vi "ex_subFileWrite.vi"(0 "Signals":dynamicdata(waveform), 1 "error in (no error)":errorcluster, 3 "Comment":string, 4 "Enable":bool=TRUE, 6 "new_file":bool, 7 "File Path in":path=path "c:/testdata.txt", 8 "File Dialog":bool, 9 "column headings":enum32{"one per segment", "once", "none"}(radio), 10 "Description":string, 11 "x_columns":enum32{"none", "one", "multiple"}(radio)=enum."multiple", 12 "multi_file":bool, 13 "fixed_width":bool=TRUE, 14 "serno_digits":i32=3, 15 "time_format_string":string="%Y-%m-%d_%H%M%S", 16 "overwrite_mode_multi":T6(ring)=enum."overwrite & backup", 17 "new_file_mode":u16(ring)=1 items=["Date & Time", "Serial No.", "Both"], 18 "overwrite_mode":T1(radio)=enum."overwrite & backup", 19 "new file options":T5, 20 "delimiter":string="\t", 22 "Reset":bool, 23 "Static File Path in":path=path "c:/testdata.txt", 24 "Lock file":bool, 25 "Simulate Non-First Call":bool, 26 "storage_format":T2, 27 "Ask each iteration":bool) -> (2 "error out":errorcluster, 5 "File Path out":path, 21 "Saving Data":bool)   [LabVIEW 2020]
uses:
  ex_NewFileOptions.ctl
  ex_WriteFileParams.ctl
  express input/ExFileReadBlock.llb/ex_ReadFileParams.ctl
  express shared/ExFile.llb/ex_FileFormats.ctl
panel:
  out "previous path":path
  in  "file params":T3={"delimiter"="\t", "origin time"=timestamp(0 s since 1904-01-01), "Flags"={"include col headings?"=TRUE, "x_columns"=0, "col headings always?"=TRUE, "time preference"=0, "hide col headings"=FALSE}, "Decimal Separator"=""} {"Flags"."time preference" items=["Absolute", "Relative"]; "Flags"."x_columns" items=["None", "One", "Multiple"]; "origin time" format="%<%X\n%x>T"}
  in  "1st":bool
  in  "File refnum":refnum<file>
  in  "origin time":timestamp format="%<%I:%M:%S %p\n%m/%d/%Y>T"
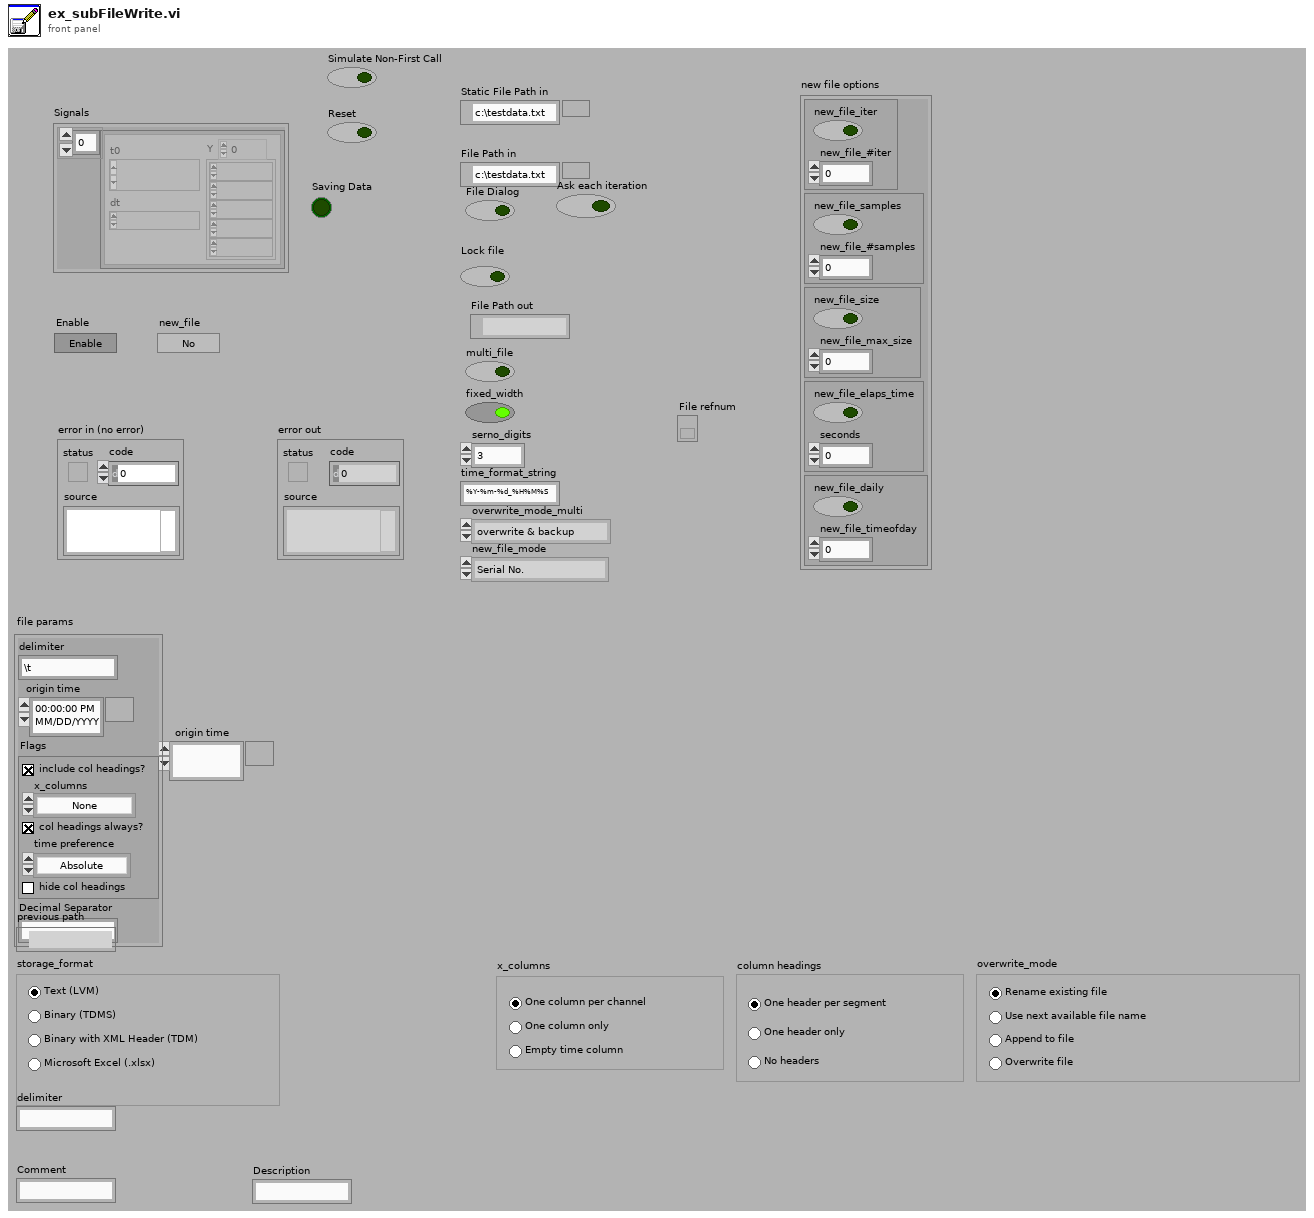
[diagram p1: front panel]
types:
  T1 = enum32{"overwrite", "overwrite & backup", "append", "next avail"}
  T2 = typedef "ex_FileFormats.ctl" = enum32{"lvm", "tdm", "tdms", "xlsx"}
  T3 = typedef "ex_WriteFileParams.ctl" = cluster{"delimiter":string, "origin time":timestamp, "Flags":T4, "Decimal Separator":string}
  T4 = typedef "ex_ReadFileParams.ctl" = cluster{"include col headings?":bool, "x_columns":u16, "col headings always?":bool, "time preference":u16, "hide col headings":bool}
  T5 = typedef "ex_NewFileOptions.ctl" = cluster{cluster{"new_file_iter":bool, "new_file_#iter":i32}, cluster{"new_file_samples":bool, "new_file_#samples":i32}, cluster{"new_file_size":bool, "new_file_max_size":i32}, cluster{"new_file_elaps_time":bool, "seconds":i32}, cluster{"new_file_daily":bool, "new_file_timeofday":i32}}
  T6 = enum16{"overwrite", "overwrite & backup", "next avail"}
  T7 = typedef "ex_userdefproperties.ctl" = cluster{"DAQmx Task":refnum<k21>, "User-defined properties":T8[], "Live values":variant[]}
  T8 = typedef "ex_userDefProperty.ctl" = cluster{"Name":string, "Object type":string, "usiDataType":T9, "propertySourceType":T10, "propertySource":string, "Value":variant, "ID":i32, "use def name":bool, "Source":string, "Built-in Prop":bool, "Attribute Type Enum":string[]}
  T9 = typedef "usiDataType.ctl" = enum16{"eNoTypeUsi", "eInt8Usi", "eInt16Usi", "eInt32Usi", "eInt64Usi", "eUInt8Usi", "eUInt16Usi", "eUInt32Usi", "eUInt64Usi", "eFloat32Usi", "eFloat64Usi", "- 0", "- 1", "- 2", "- 3", "- 4", "- 5", "- 6", "- 7", "- 8", "- 9", "eString8Usi", "eString16Usi", "eStringUsi", "eEnumUsi", "- 10", "- 11", "- 12", "- 13", "- 14", "eTimeUsi", "- 15", "- 16", "- 17", "- 18", "- 19", "- 20", "- 21", "- 22", "- 23", "eInstanceUsi", "eStoreUsi"}
  T10 = typedef "ex_propertySource.ctl" = enum16{"Manual", "System", "DAQmx Channel", "Terminal", "Ignore"}
  T11 = cluster{"file params":T3, "column headings":enum32{"one per segment", "once", "none"}, "origin time":timestamp, "File refnum":refnum<file>, "overwrite_mode_multi":enum16{"overwrite", "overwrite & backup", "next avail"}, "overwrite_mode":enum32{"overwrite", "overwrite & backup", "append", "next avail"}, "File Dialog":bool, "Description Out":string, "Comment Out":string, "serno_digits":i32, "fixed_width":bool, "new_file_mode":u16, "time_format_string":string, "multi_file":bool, "new file options":T5, "new_file":bool, "Simulate Non-First Call":bool}
  T12 = cluster{"channel\nrefnums":refnum<k20>[], "channel names":string[], "channel types":string[], "file refnum":refnum<k20>, "group refnum":refnum<k20>, "group name":string, "group type":string, "next T0":timestamp[], "dT":dbl[], "Start Time Stamp":timestamp, "channel length":u32[], "group index":u32, "group refnums":refnum<k20>[], "file name":string, "segment index":u32}
  T13 = typedef "ex_appendInfoTDM.ctl" = cluster{"channel\nrefnums":refnum<k20>[], "channel names":string[], "channel types":string[], "file refnum":refnum<k20>, "group refnum":refnum<k20>, "group name":string, "group type":string, "next T0":timestamp[], "dT":dbl[], "Start Time Stamp":timestamp, "channel length":u32[], "group index":u32, "group refnums":refnum<k20>[], "file name":string, "segment index":u32}
  T14 = cluster{"Start Timestamp":timestamp, "Timestamp":timestamp, "Relative Time?":bool, "X Dimension":string, "Signal Name":string, "Y Units":string, "X0":timestamp, "dX":dbl, "nPoints":i32}[]
  T15 = typedef "ex_WaveformAttribsPlus.ctl" = cluster{"Start Timestamp":timestamp, "Timestamp":timestamp, "Relative Time?":bool, "X Dimension":string, "Signal Name":string, "Y Units":string, "X0":timestamp, "dX":dbl, "nPoints":i32}
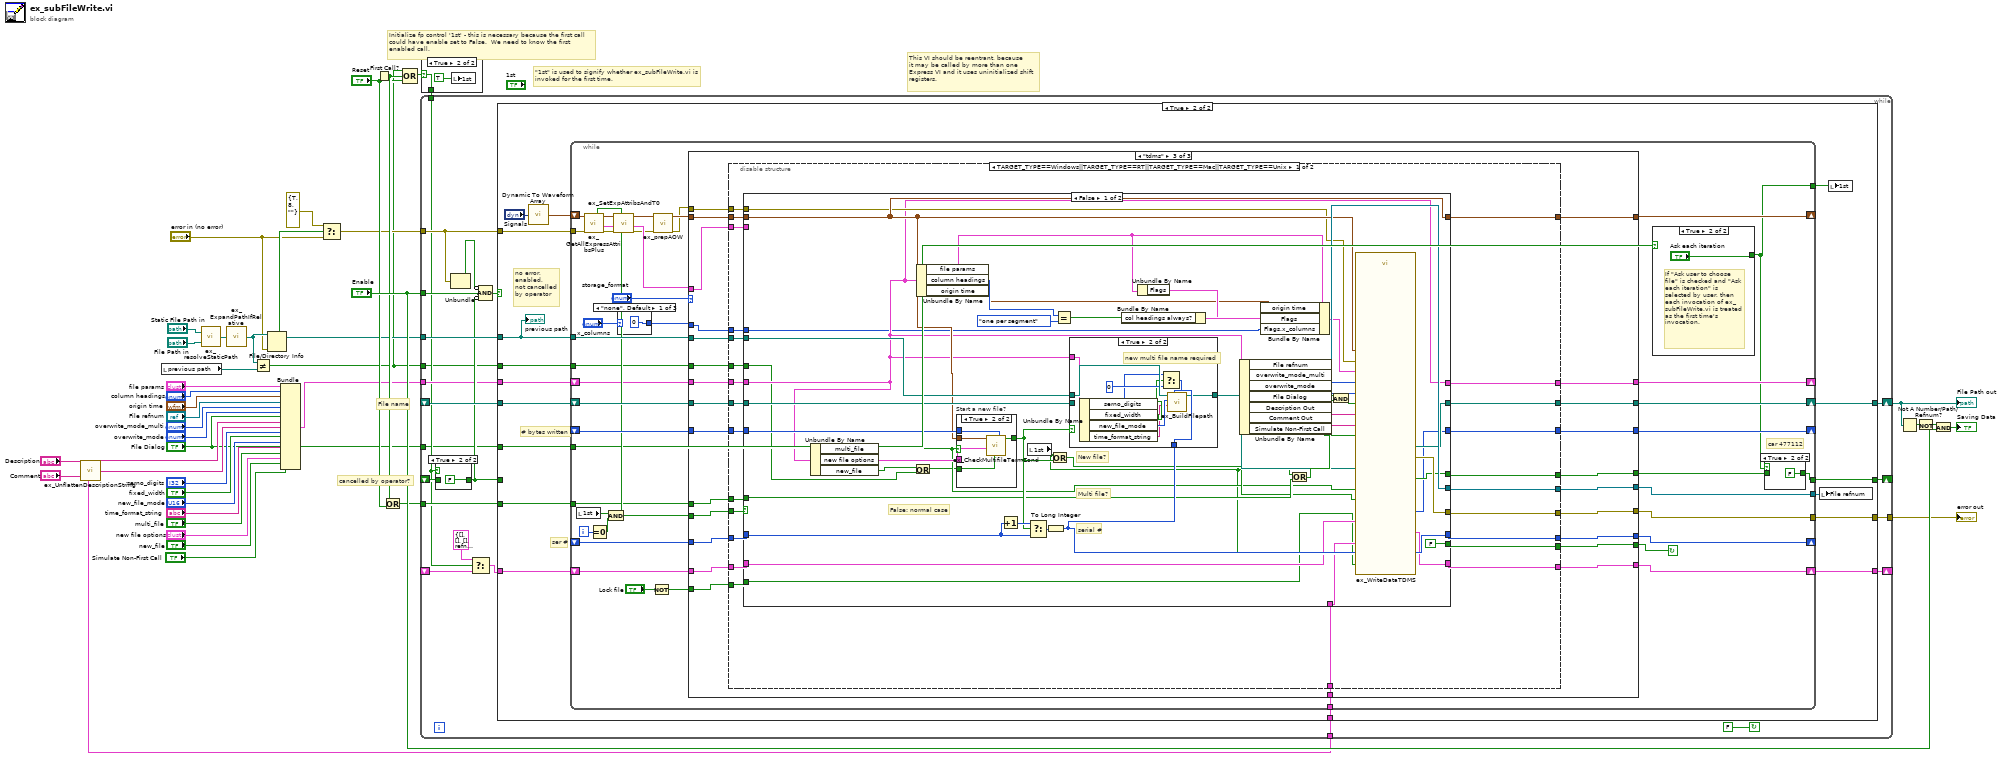
[diagram p0: block diagram]
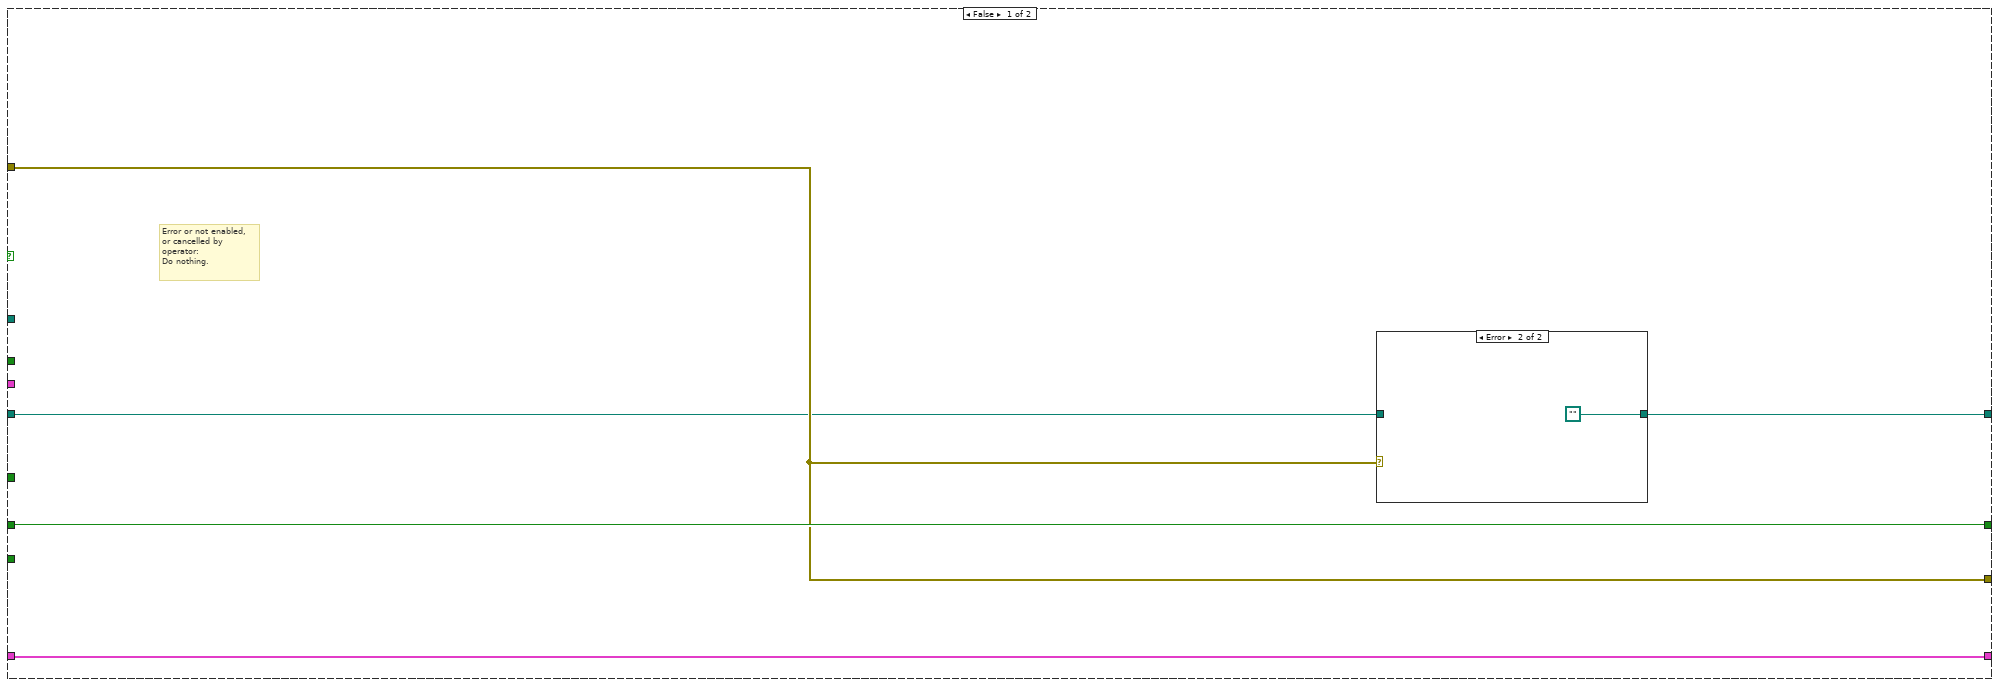
[diagram p3: hidden frame]
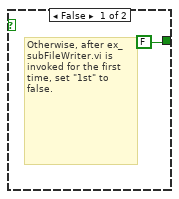
[diagram p6: hidden frame]
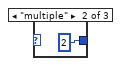
[diagram p7: hidden frame]
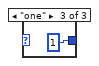
[diagram p8: hidden frame]
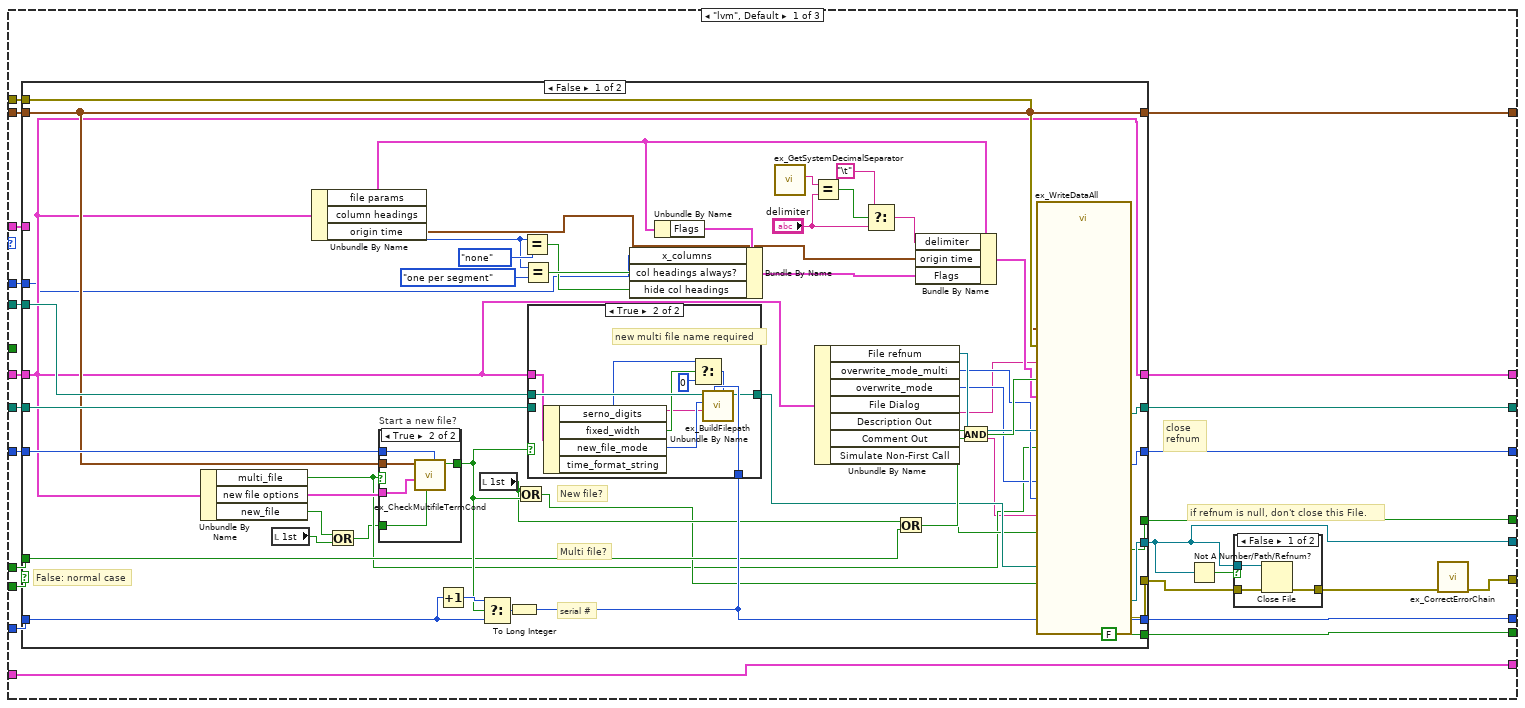
[diagram p9: hidden frame]
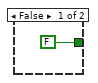
[diagram p12: hidden frame]
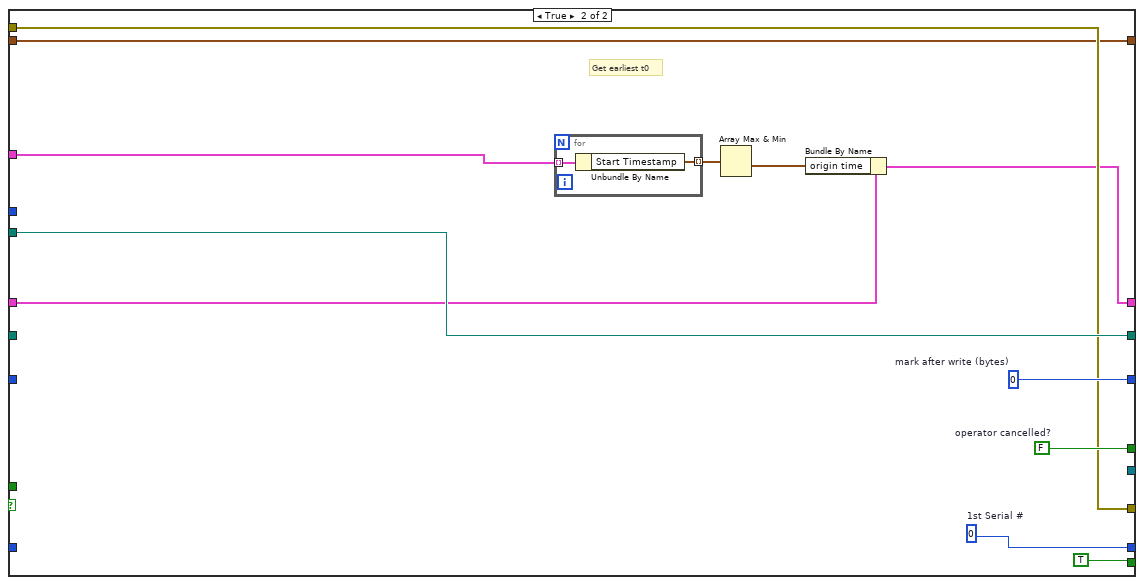
[diagram p13: hidden frame]
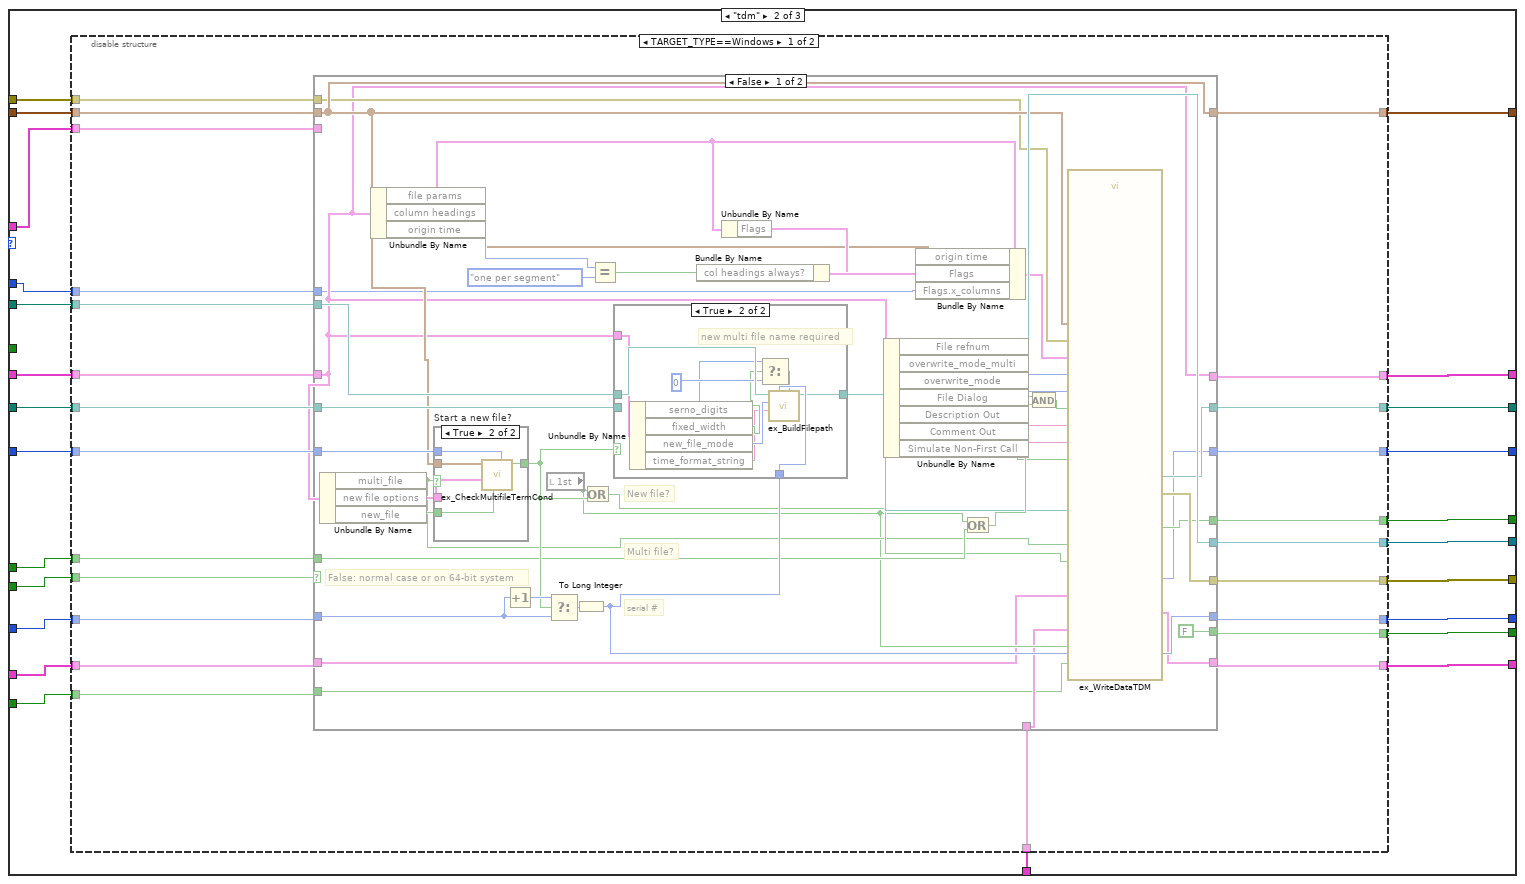
[diagram p14: hidden frame]
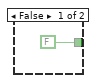
[diagram p16: hidden frame]
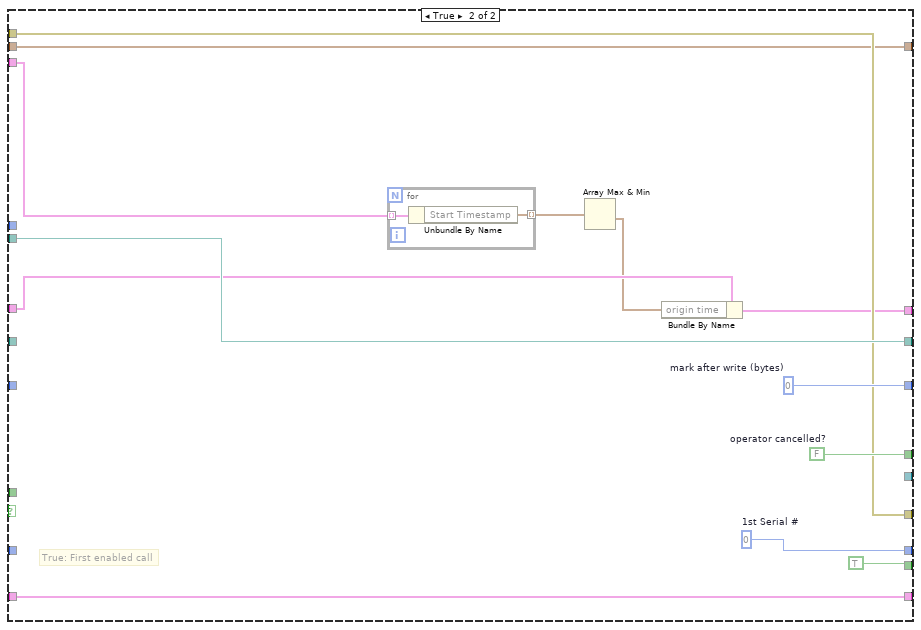
[diagram p17: hidden frame]
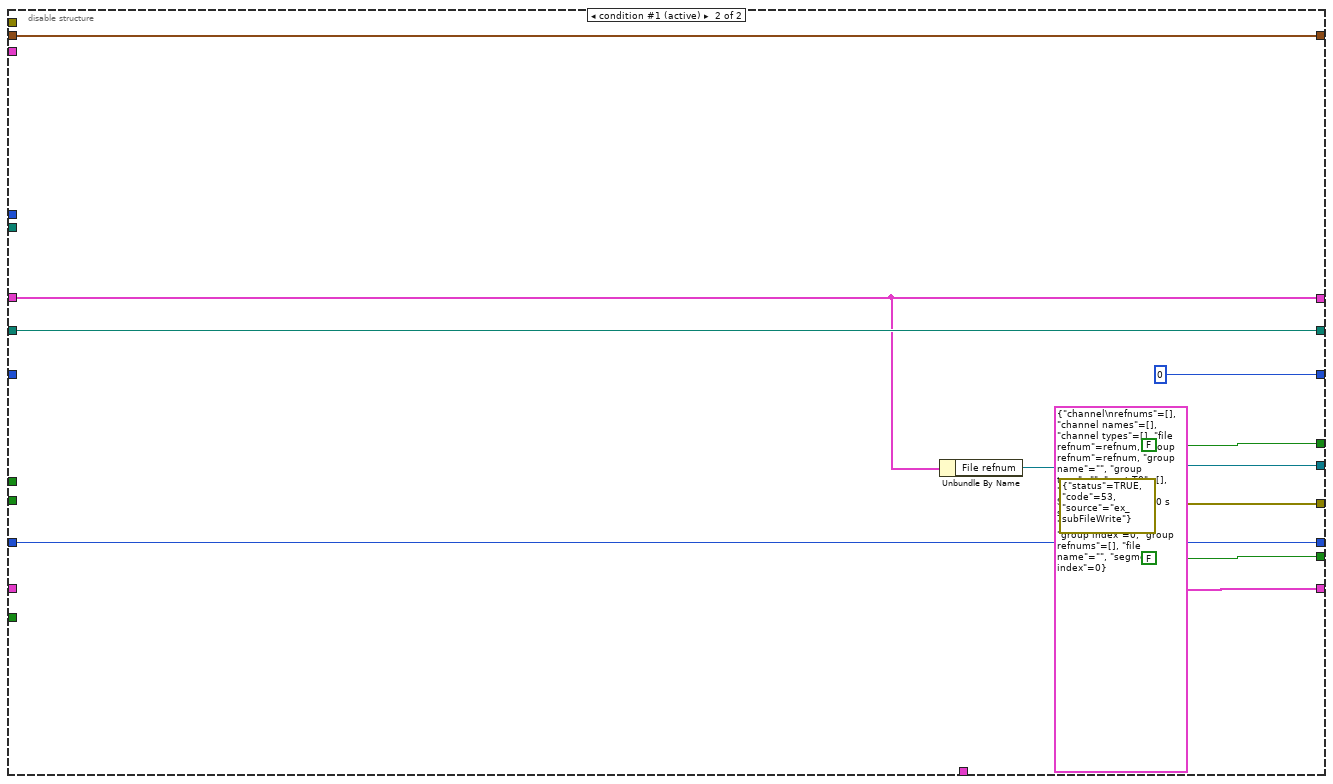
[diagram p18: hidden frame]
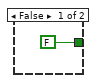
[diagram p20: hidden frame]
diagram:
  # "\"1st\" is used to signify whether ex_subFileWrite.vi is invoked for the first time."
  # "File name"
  # "This VI should be reentrant, because\nit may be called by more than one\nExpress VI and it uses uninitialized shift \nregisters."
  # "cancelled by operator?"
  # "Initialize fp control '1st' - this is necessary because the first call\ncould have enable set to False.  We need to know the first\nenabled call."
  n1 = call "ex_UnflattenDescriptionString.vi"("Description"="Description", "Comment"="Comment") -> ("Description Out"=w7:string, "Comment Out"=w6:string, "DAQmx Task"=w5:T7)
  n2 = local read "previous path"() -> (w36:path)
  n3 = call "ex_resolveStaticPath.vi"("file path in"="File Path in", "static path in"="Static File Path in") -> ("Path"=w14:path)
  n4 = call "ex_ExpandPathIfRelative.vi"("Path"=w14) -> ("Expanded path"=w13:path)  [unwired: 4 out]
  n5 = Not Equal?(x=w13, y=w36) -> (x != y?=w1:bool)
  n6 = File/Directory Info(path=w13, error in="error in (no error)") -> (path out=w12:path, directory=w10:bool)  [unwired: 5 out]
  n7 = Bundle("file params"="file params", "column headings"="column headings", "origin time"="origin time", "File refnum"="File refnum", "overwrite_mode_multi"="overwrite_mode_multi", "overwrite_mode"="overwrite_mode", "File Dialog"="File Dialog", "Description Out"=w7, "Comment Out"=w6, "serno_digits"="serno_digits", "fixed_width"="fixed_width", "new_file_mode"="new_file_mode", "time_format_string"="time_format_string", "multi_file"="multi_file", "new file options"="new file options", "new_file"="new_file", "Simulate Non-First Call"="Simulate Non-First Call") -> (w15:T11)  [unwired: 1 out]
  n8 = Select(t=errorcluster {"status"=TRUE, "code"=8, "source"=""}, s=w10, f="error in (no error)") -> (s? t:f=w11:errorcluster)
  n9 = First Call?() -> (First Call?: T/F=w34:bool)
  n10 = Or(x=w34, y="Reset") -> (x .or. y?=w32:bool)
  n11 = Compound Arithmetic op=OR(w1, w34, "Reset") -> (w35:bool)
  n12 = case shown="True" w35 {
    selector: w35 -> [w44 w45]
    tunnel: [w44 w45] -> w43
    frame False {
    }
    frame True {
      n13 = local write "1st"(TRUE ("1st")) -> ()
    }
  }
  n14 = while {
    tunnel: [w68] -> w31
    tunnel: w43 -> [w49]
    tunnel: w11 -> [w66]
    shift-right: [w64] -> _
    shift-left: _ -> [w63]
    shift-right: [w61] -> w30
    shift-left: _ -> [w62]
    tunnel: "Enable" -> [w60]
    tunnel: w12 -> [w59]
    tunnel: w32 -> [w56]
    tunnel: w15 -> [w55]
    shift-right: [w54] -> _
    shift-left: _ -> [w51]
    tunnel: w5 -> [w53]
    tunnel: "File Dialog" -> [w48]
    tunnel: w1 -> [w47]
    stop <- FALSE continue-if-true
    n15 = case shown="True" w49 {
      tunnel: w63 -> [w69 _]
      tunnel: [w69 FALSE ("operator cancelled?")] -> w57
      frame False {
      }
      frame True {
      }
    }
    n16 = Unbundle(w66) -> ("status"=w58:bool)  [unwired: 2 out]
    n17 = Select(t=T12 {"channel\nrefnums"=[], "channel names"=[], "channel types"=[], "file refnum"=refnum, "group refnum"=refnum, "group name"="", "group type"="", "next T0"=[], "dT"=[], "Start Time Stamp"=timestamp(0 s since 1904-01-01), "channel length"=[], "group index"=0, "group refnums"=[], "file name"="", "segment index"=0} ("append info out"), s=w49, f=w51) -> (s? t:f=w50:T13)
    n18 = Compound Arithmetic op=AND(invert w58, w60, invert w57) -> (w67:bool)
    n19 = case shown="True" w67 {
      tunnel: [w73 w85] -> w68
      tunnel: w66 -> [w73 w94]
      tunnel: [w75 w93] -> w64
      tunnel: w57 -> [w75 _]
      tunnel: [w72 w92] -> w61
      tunnel: w62 -> [w71 w91]
      tunnel: w59 -> [_ w82]
      tunnel: w56 -> [_ w89]
      tunnel: w55 -> [_ w87]
      tunnel: [w74 w84] -> w54
      tunnel: w50 -> [w74 w83]
      tunnel: w53 -> [_ w81]
      tunnel: w48 -> [_ w79]
      tunnel: w47 -> [_ w78]
      frame False {
        # "Error or not enabled,\nor cancelled by\noperator:\nDo nothing."
        n20 = case shown="Error" w73 {
          tunnel: [w76 path ""] -> w72
          tunnel: w71 -> [w76 _]
          frame No Error {
          }
          frame Error {
          }
        }
      }
      frame True {
        # "no error,\nenabled,\nnot cancelled\nby operator"
        # "# bytes written"
        # "ser #"
        n21 = call "Dynamic To Waveform Array.vi"("Input"="Signals") -> ("Output"=w86:waveform(dbl)[])  [unwired: 4 out]
        n22 = while {
          tunnel: w94 -> [w124]
          shift-right: [w133] -> _
          shift-left: _ -> [w132]
          tunnel: [w135] -> w85
          shift-right: [w125] -> w92
          shift-left: w91 -> [w131]
          shift-right: [w127] -> _
          shift-left: _ -> [w134]
          tunnel: [w130] -> w88
          tunnel: w82 -> [w126]
          tunnel: [w96] -> w93
          shift-right: [w123] -> _
          shift-left: w86 -> [w112]
          tunnel: w89 -> [w115]
          shift-right: [w111] -> _
          shift-left: w87 -> [w113]
          shift-right: [w110] -> w84
          shift-left: w83 -> [w109]
          tunnel: w81 -> [w102]
          tunnel: [w98] -> w80
          tunnel: w79 -> [w99]
          tunnel: w78 -> [w95]
          i -> [w129]
          stop <- w136 continue-if-true
          # "car 477112"
          n23 = local read "1st"() -> (w116:bool)
          n24 = call "ex_GetAllExpressAttribsPlus.vi"("error in"=w124, "Signals in"=w112) -> ("error out"=w118:errorcluster, "All Express Wave Attributes Plus"=w117:T14, "Signals out"=w121:waveform(dbl)[], "Time Attribs Not Found"=w119:bool[])  [unwired: 1 in, 5 out]
          n25 = Equal To 0?(x=w129) -> (x = 0?=w128:bool)
          n26 = And(x=w116, y=w128) -> (x .and. y?=w122:bool)
          n27 = call "ex_SetExpAttribsAndT0.vi"("Latch Origin TS? (T)"=w122, "Set? (T if empty)"=w119, "error in (no error)"=w118, "Express Attributes Plus in"=w117, "Signals"=w121) -> ("error out"=w104:errorcluster, "Express Wave Attributes Plus out"=w120:T15[], "Signals With Attributes"=w106:waveform(dbl)[])  [unwired: 1 in, 3 out]
          n28 = case shown="\"none\", Default" "x_columns" {
            tunnel: [u16 0 ("x_columns") u16 2 ("x_columns") u16 1 ("x_columns")] -> w107
            frame "none", Default {
            }
            frame "multiple" {
            }
            frame "one" {
            }
          }
          n29 = Not(x="Lock file") -> (.not. x?=w100:bool)
          n30 = call "ex_prepAOW.vi"("error in (no error)"=w104, "Dynamic Data"=w106) -> ("error out"=w103:errorcluster, 3:w105:waveform(dbl)[])  [unwired: 1 in, 3 out]
          n31 = case shown="\"tdms\"" "storage_format" {
            tunnel: [w167 w277 w413] -> w136
            tunnel: [w151 w276 w412] -> w135
            tunnel: w134 -> [w166 w275 w411]
            tunnel: [w165 w274 w410] -> w133
            tunnel: w132 -> [w164 w273 w409]
            tunnel: w131 -> [w163 w272 w408]
            tunnel: [w144 w261 w397] -> w130
            tunnel: [w162 w271 w407] -> w127
            tunnel: w126 -> [w161 w270 w406]
            tunnel: [w160 w269 w405] -> w97
            tunnel: [w159 w268 w404] -> w125
            tunnel: [w158 w267 w403] -> w123
            tunnel: w122 -> [w157 w266 w402]
            tunnel: w105 -> [w156 w260 w396]
            tunnel: w103 -> [w155 w265 w401]
            tunnel: w120 -> [w154 w264 w400]
            tunnel: w115 -> [w153 w263 w399]
            tunnel: w113 -> [w152 w262 w398]
            tunnel: [w150 w259 w395] -> w111
            tunnel: [w149 w258 w394] -> w110
            tunnel: w109 -> [w149 w257 w393]
            tunnel: w107 -> [w148 w256 w392]
            tunnel: w102 -> [_ w255 w391]
            tunnel: w100 -> [_ w254 w390]
            tunnel: w95 -> [_ _ w389]
            frame "lvm", Default {
              # "if refnum is null, don't close this File."
              # "close\nrefnum"
              n32 = case shown="False" w157 {
                tunnel: [FALSE TRUE] -> w167
                tunnel: [w195 _] -> w144
                tunnel: [w192 w244] -> w147
                tunnel: [w193 w251] -> w162
                tunnel: w166 -> [w215 _]
                tunnel: w155 -> [w211 w244]
                tunnel: [w220 w249] -> w165
                tunnel: [w194 w250] -> w159
                tunnel: w164 -> [w221 _]
                tunnel: w163 -> [w217 _]
                tunnel: w156 -> [w185 w243]
                tunnel: w161 -> [w214 w250]
                tunnel: [w186 w247] -> w160
                tunnel: w154 -> [_ w245]
                tunnel: [w185 w243] -> w158
                tunnel: w153 -> [w204 _]
                tunnel: w152 -> [w183 w242]
                tunnel: [w183 w240] -> w150
                tunnel: w148 -> [w182 _]
                frame False {
                  # "Multi file?"
                  # "New file?"
                  # "False: normal case"
                  # "serial #"
                  n33 = Unbundle By Name(w183) -> ("multi_file"=w187:bool, "new file options"=w196:T5, "new_file"=w174:bool)
                  n34 = local read "1st"() -> (w173:bool)
                  n35 = Unbundle By Name(w183) -> ("file params"=w202:T3, "column headings"=w201:enum32{"one per segment", "once", "none"}, "origin time"=w184:timestamp)
                  n36 = Or(x=w174, y=w173) -> (x .or. y?=w172:bool)
                  n37 = case "Start a new file?" shown="True" w187 {
                    tunnel: [FALSE ("start new file?") w239] -> w216
                    tunnel: w185 -> [_ w238]
                    tunnel: w215 -> [_ w237]
                    tunnel: w196 -> [_ w236]
                    tunnel: w172 -> [_ w235]
                    frame False {
                    }
                    frame True {
                      n38 = call "ex_CheckMultifileTermCond.vi"("file size (bytes)"=w237, "new_file_now"=w235, "termination conditions"=w236, "Signals"=w238) -> ("start new file?"=w239:bool)  [unwired: 7 out]
                    }
                  }
                  n39 = Increment(x=w221) -> (x+1=w222:i32)
                  n40 = local read "1st"() -> (w203:bool)
                  n41 = Select(t=w222, s=w216, f=w221) -> (s? t:f=w219:i32)
                  n42 = To Long Integer(number=w219) -> (32bit integer=w220:i32)
                  n43 = Or(x=w203, y=w216) -> (x .or. y?=w188:bool)
                  n44 = Equal?(x=w201, y=enum16{"one per segment", "once", "none"}."none") -> (x = y?=w207:bool)
                  n45 = Equal?(x=w201, y=enum16{"one per segment", "once", "none"}."one per segment") -> (x = y?=w208:bool)
                  n46 = case shown="True" w216 {
                    tunnel: w220 -> [_ w233]
                    tunnel: [w223 w232] -> w191
                    tunnel: w217 -> [w223 _]
                    tunnel: w214 -> [_ w231]
                    tunnel: w183 -> [_ w228]
                    frame False {
                      # "No new file - use old file name"
                    }
                    frame True {
                      # "new multi file name required"
                      n47 = Unbundle By Name(w228) -> ("serno_digits"=w227:i32, "fixed_width"=w226:bool, "new_file_mode"=w225:u16, "time_format_string"=w224:string)
                      n48 = Select(t=w227, s=w226, f=0) -> (s? t:f=w229:i32)
                      n49 = call "ex_BuildFilepath.vi"("serial digits"=w229, "serial num"=w233, "time format string"=w224, "naming mode"=w225, "name base"=w231) -> ("built name"=w232:path)  [unwired: 1 in, 5 out]
                    }
                  }
                  n50 = Unbundle By Name(w202) -> ("Flags"=w212:T4)
                  n51 = Bundle By Name(cluster=w212, "x_columns"=w182, "col headings always?"=w208, "hide col headings"=w207) -> (w213:T4)
                  n52 = call "ex_GetSystemDecimalSeparator.vi"() -> ("Decimal Seperator"=w179:string)  [unwired: 11 out]
                  n53 = Equal?(x=w179, y="delimiter") -> (x = y?=w178:bool)
                  n54 = Unbundle By Name(w183) -> ("File refnum"=w200:refnum<file>, "overwrite_mode_multi"=w199:T6, "overwrite_mode"=w198:T1, "File Dialog"=w197:bool, "Description Out"=w180:string, "Comment Out"=w181:string, "Simulate Non-First Call"=w190:bool)
                  n55 = Select(t="\t", s=w178, f="delimiter") -> (s? t:f=w175:string)
                  n56 = Or(x=w203, y=w204) -> (x .or. y?=w206:bool)
                  n57 = Bundle By Name(cluster=w202, "delimiter"=w175, "origin time"=w184, "Flags"=w213) -> (w189:T3)
                  n58 = And(x=w197, y=w206) -> (x .and. y?=w205:bool)
                  n59 = call "ex_WriteDataAll.vi"("file path"=w191, "File refnum in"=w200, "Signals"=w185, "overwrite_mode_multi"=w199, "overwrite_mode"=w198, "error in (no error)"=w211, "file dialog?"=w205, "Description"=w180, "multi_file"=w187, "Comment"=w181, "new file?"=w188, "Simulate Non-First Call"=w190, "file params"=w189) -> ("operator cancelled?"=w186:bool, "file path out"=w194:path, "refnum out"=w195:refnum<file>, "mark after write (bytes)"=w193:i32, "error out"=w192:errorcluster)  [unwired: 2 out]
                }
                frame True {
                  w247 = FALSE  # operator cancelled?
                  w251 = 0  # mark after write (bytes)
                  w249 = 0  # 1st Serial #
                  # "True: First enabled call"
                  # "Get earliest t0"
                  n60 = for {
                    tunnel: w245 -> [w253] mode=indexing
                    tunnel: [w252] -> w246 mode=indexing
                    n61 = Unbundle By Name(w253) -> ("Start Timestamp"=w252:timestamp)
                  }
                  n62 = Array Max & Min(array=w246) -> (min value=w241:timestamp)  [unwired: 3 out]
                  n63 = Bundle By Name(cluster=w242, "origin time"=w241) -> (w240:T11)
                }
              }
              n64 = Not A Number/Path/Refnum?(number/path/refnum=w144) -> (NaN/Path/Refnum?=w145:bool)
              n65 = case shown="False" w145 {
                tunnel: w147 -> [w170 w171]
                tunnel: [w169 w171] -> w146
                tunnel: w144 -> [w168 _]
                frame False {
                  n66 = Close File(refnum=w168, error in=w170) -> (error out=w169:errorcluster)  [unwired: 1 out]
                }
                frame True {
                }
              }
              n67 = call "ex_CorrectErrorChain.vi"("error in (no error)"=w146) -> ("error out"=w151:errorcluster)  [unwired: 1 in, 9 out]
            }
            frame "tdm" {
              n68 = disable-structure shown="TARGET_TYPE==Windows" {
                disable-tunnel: [w301 FALSE] -> w277
                disable-tunnel: [w300 errorcluster {"status"=TRUE, "code"=53, "source"="ex_subFileWrite"} ("error out")] -> w276
                disable-tunnel: w275 -> [w299 _]
                disable-tunnel: [w298 w383] -> w274
                disable-tunnel: w273 -> [w297 w383]
                disable-tunnel: w272 -> [w296 w388]
                disable-tunnel: [w295 0 ("mark after write (bytes)")] -> w271
                disable-tunnel: w270 -> [w294 _]
                disable-tunnel: [w293 FALSE ("operator cancelled?")] -> w269
                disable-tunnel: [w292 w388] -> w268
                disable-tunnel: [w291 w387] -> w267
                disable-tunnel: w266 -> [w278 _]
                disable-tunnel: w265 -> [w290 _]
                disable-tunnel: w264 -> [w289 _]
                disable-tunnel: w263 -> [w279 _]
                disable-tunnel: w262 -> [w288 w386]
                disable-tunnel: [w287 w385] -> w261
                disable-tunnel: w260 -> [w286 w387]
                disable-tunnel: [w285 w386] -> w259
                disable-tunnel: [w284 T12 {"channel\nrefnums"=[], "channel names"=[], "channel types"=[], "file refnum"=refnum, "group refnum"=refnum, "group name"="", "group type"="", "next T0"=[], "dT"=[], "Start Time Stamp"=timestamp(0 s since 1904-01-01), "channel length"=[], "group index"=0, "group refnums"=[], "file name"="", "segment index"=0} ("append info out")] -> w258
                disable-tunnel: w257 -> [w283 _]
                disable-tunnel: w256 -> [w282 _]
                disable-tunnel: w255 -> [w281 _]
                disable-tunnel: w254 -> [w280 _]
                frame condition #0 {
                  n69 = case shown="False" w278 {
                    tunnel: [FALSE TRUE] -> w301
                    tunnel: [w311 w371] -> w300
                    tunnel: [w309 w376] -> w295
                    tunnel: w299 -> [w339 _]
                    tunnel: w290 -> [w324 w371]
                    tunnel: [w344 w374] -> w298
                    tunnel: [w312 w375] -> w292
                    tunnel: w297 -> [w345 _]
                    tunnel: w296 -> [w341 _]
                    tunnel: w294 -> [w338 w375]
                    tunnel: [w310 w372] -> w293
                    tunnel: w289 -> [_ w369]
                    tunnel: [w325 w370] -> w291
                    tunnel: w279 -> [w332 _]
                    tunnel: w288 -> [w322 w367]
                    tunnel: [w326 _] -> w287
                    tunnel: w286 -> [w325 w370]
                    tunnel: [w322 w365] -> w285
                    tunnel: [w308 w364] -> w284
                    tunnel: w283 -> [w307 w364]
                    tunnel: w282 -> [w321 _]
                    tunnel: w281 -> [w306 _]
                    tunnel: w280 -> [w302 _]
                    frame False {
                      # "Multi file?"
                      # "New file?"
                      # "False: normal case or on 64-bit system"
                      # "serial #"
                      n70 = Unbundle By Name(w322) -> ("multi_file"=w314:bool, "new file options"=w328:T5, "new_file"=w327:bool)
                      n71 = Unbundle By Name(w322) -> ("file params"=w331:T3, "column headings"=w330:enum32{"one per segment", "once", "none"}, "origin time"=w323:timestamp)
                      n72 = case "Start a new file?" shown="True" w314 {
                        tunnel: [FALSE ("start new file?") w363] -> w340
                        tunnel: w325 -> [_ w362]
                        tunnel: w339 -> [_ w361]
                        tunnel: w328 -> [_ w360]
                        tunnel: w327 -> [_ w359]
                        frame False {
                        }
                        frame True {
                          n73 = call "ex_CheckMultifileTermCond.vi"("file size (bytes)"=w361, "new_file_now"=w359, "termination conditions"=w360, "Signals"=w362) -> ("start new file?"=w363:bool)  [unwired: 7 out]
                        }
                      }
                      n74 = Increment(x=w345) -> (x+1=w346:i32)
                      n75 = local read "1st"() -> (w313:bool)
                      n76 = Select(t=w346, s=w340, f=w345) -> (s? t:f=w343:i32)
                      n77 = To Long Integer(number=w343) -> (32bit integer=w344:i32)
                      n78 = Or(x=w313, y=w340) -> (x .or. y?=w315:bool)
                      n79 = Equal?(x=w330, y=enum16{"one per segment", "once", "none"}."one per segment") -> (x = y?=w334:bool)
                      n80 = case shown="True" w340 {
                        tunnel: w344 -> [_ w357]
                        tunnel: [w347 w356] -> w316
                        tunnel: w341 -> [w347 _]
                        tunnel: w338 -> [_ w355]
                        tunnel: w322 -> [_ w352]
                        frame False {
                          # "No new file - use old file name"
                        }
                        frame True {
                          # "new multi file name required"
                          n81 = Unbundle By Name(w352) -> ("serno_digits"=w351:i32, "fixed_width"=w350:bool, "new_file_mode"=w349:u16, "time_format_string"=w348:string)
                          n82 = Select(t=w351, s=w350, f=0) -> (s? t:f=w353:i32)
                          n83 = call "ex_BuildFilepath.vi"("serial digits"=w353, "serial num"=w357, "time format string"=w348, "naming mode"=w349, "name base"=w355) -> ("built name"=w356:path)  [unwired: 1 in, 5 out]
                        }
                      }
                      n84 = Unbundle By Name(w331) -> ("Flags"=w336:T4)
                      n85 = Bundle By Name(cluster=w336, "col headings always?"=w334) -> (w337:T4)
                      n86 = Unbundle By Name(w322) -> ("File refnum"=w326:refnum<file>, "overwrite_mode_multi"=w319:T6, "overwrite_mode"=w318:T1, "File Dialog"=w329:bool, "Description Out"=w304:string, "Comment Out"=w303:string, "Simulate Non-First Call"=w305:bool)
                      n87 = Bundle By Name(cluster=w331, "origin time"=w323, "Flags"=w337, "Flags.x_columns"=w321) -> (w320:T3)
                      n88 = Or(x=w313, y=w332) -> (x .or. y?=w333:bool)
                      n89 = And(x=w329, y=w333) -> (x .and. y?=w317:bool)
                      n90 = call "ex_WriteDataTDM.vi"("file path"=w316, "first call"=w313, "Lock file"=w302, "Signals"=w325, "overwrite_mode_multi"=w319, "overwrite_mode"=w318, "error in (no error)"=w324, "file dialog?"=w317, "Description"=w304, "multi_file"=w314, "Comment"=w303, "new file?"=w315, "Simulate Non-First Call"=w305, "file params"=w320, "append info"=w307, "DAQmx Task"=w306) -> ("operator cancelled?"=w310:bool, "file path out"=w312:path, "bytes written"=w309:i32, "append info out"=w308:T13, "error out"=w311:errorcluster)  [unwired: 7 out]
                    }
                    frame True {
                      w372 = FALSE  # operator cancelled?
                      w376 = 0  # mark after write (bytes)
                      w374 = 0  # 1st Serial #
                      # "True: First enabled call"
                      n91 = for {
                        tunnel: w369 -> [w378] mode=indexing
                        tunnel: [w377] -> w368 mode=indexing
                        n92 = Unbundle By Name(w378) -> ("Start Timestamp"=w377:timestamp)
                      }
                      n93 = Array Max & Min(array=w368) -> (min value=w366:timestamp)  [unwired: 3 out]
                      n94 = Bundle By Name(cluster=w367, "origin time"=w366) -> (w365:T11)
                    }
                  }
                }
                frame condition #1 (active) {
                  n95 = Unbundle By Name(w386) -> ("File refnum"=w385:refnum<file>)
                }
              }
            }
            frame "tdms" {
              n96 = disable-structure shown="TARGET_TYPE==Windows||TARGET_TYPE==RT||TARGET_TYPE==Mac||TARGET_TYPE==Unix" {
                disable-tunnel: [w438 FALSE] -> w413
                disable-tunnel: [w437 errorcluster {"status"=TRUE, "code"=53, "source"="ex_subFileWrite"} ("error out")] -> w412
                disable-tunnel: w411 -> [w436 _]
                disable-tunnel: [w435 w522] -> w410
                disable-tunnel: w409 -> [w434 w522]
                disable-tunnel: w408 -> [w433 w527]
                disable-tunnel: [w432 0 ("mark after write (bytes)")] -> w407
                disable-tunnel: w406 -> [w431 _]
                disable-tunnel: [w430 FALSE ("operator cancelled?")] -> w405
                disable-tunnel: [w429 w527] -> w404
                disable-tunnel: [w428 w526] -> w403
                disable-tunnel: w402 -> [w427 _]
                disable-tunnel: w401 -> [w426 _]
                disable-tunnel: w400 -> [w425 _]
                disable-tunnel: w399 -> [w424 _]
                disable-tunnel: w398 -> [w423 w525]
                disable-tunnel: [w422 w524] -> w397
                disable-tunnel: w396 -> [w421 w526]
                disable-tunnel: [w420 w525] -> w395
                disable-tunnel: [w419 T12 {"channel\nrefnums"=[], "channel names"=[], "channel types"=[], "file refnum"=refnum, "group refnum"=refnum, "group name"="", "group type"="", "next T0"=[], "dT"=[], "Start Time Stamp"=timestamp(0 s since 1904-01-01), "channel length"=[], "group index"=0, "group refnums"=[], "file name"="", "segment index"=0} ("append info out")] -> w394
                disable-tunnel: w393 -> [w418 _]
                disable-tunnel: w392 -> [w417 _]
                disable-tunnel: w391 -> [w416 _]
                disable-tunnel: w390 -> [w415 _]
                disable-tunnel: w389 -> [w414 _]
                frame condition #0 (active) {
                  n97 = case shown="False" w427 {
                    tunnel: [FALSE TRUE] -> w438
                    tunnel: [w451 w510] -> w437
                    tunnel: [w449 w515] -> w432
                    tunnel: w436 -> [w478 _]
                    tunnel: w426 -> [w464 w510]
                    tunnel: [w483 w513] -> w435
                    tunnel: [w452 w514] -> w429
                    tunnel: w434 -> [w484 _]
                    tunnel: w433 -> [w480 _]
                    tunnel: w431 -> [w477 w514]
                    tunnel: [w450 w511] -> w430
                    tunnel: w425 -> [_ w508]
                    tunnel: [w465 w509] -> w428
                    tunnel: w424 -> [w471 _]
                    tunnel: w423 -> [w462 w506]
                    tunnel: [w466 _] -> w422
                    tunnel: w421 -> [w465 w509]
                    tunnel: [w462 w504] -> w420
                    tunnel: [w448 w503] -> w419
                    tunnel: w418 -> [w447 w503]
                    tunnel: w417 -> [w461 _]
                    tunnel: w416 -> [w446 _]
                    tunnel: w415 -> [w442 _]
                    tunnel: w414 -> [w439 _]
                    frame False {
                      # "Multi file?"
                      # "New file?"
                      # "False: normal case"
                      # "serial #"
                      n98 = Unbundle By Name(w462) -> ("multi_file"=w454:bool, "new file options"=w467:T5, "new_file"=w441:bool)
                      n99 = Or(x=w441, y=w439) -> (x .or. y?=w440:bool)
                      n100 = Unbundle By Name(w462) -> ("file params"=w470:T3, "column headings"=w469:enum32{"one per segment", "once", "none"}, "origin time"=w463:timestamp)
                      n101 = case "Start a new file?" shown="True" w454 {
                        tunnel: [FALSE ("start new file?") w502] -> w479
                        tunnel: w465 -> [_ w501]
                        tunnel: w478 -> [_ w500]
                        tunnel: w467 -> [_ w499]
                        tunnel: w440 -> [_ w498]
                        frame False {
                        }
                        frame True {
                          n102 = call "ex_CheckMultifileTermCond.vi"("file size (bytes)"=w500, "new_file_now"=w498, "termination conditions"=w499, "Signals"=w501) -> ("start new file?"=w502:bool)  [unwired: 7 out]
                        }
                      }
                      n103 = Increment(x=w484) -> (x+1=w485:i32)
                      n104 = local read "1st"() -> (w453:bool)
                      n105 = Select(t=w485, s=w479, f=w484) -> (s? t:f=w482:i32)
                      n106 = To Long Integer(number=w482) -> (32bit integer=w483:i32)
                      n107 = Or(x=w453, y=w479) -> (x .or. y?=w455:bool)
                      n108 = Equal?(x=w469, y=enum16{"one per segment", "once", "none"}."one per segment") -> (x = y?=w473:bool)
                      n109 = case shown="True" w479 {
                        tunnel: w483 -> [_ w496]
                        tunnel: [w486 w495] -> w456
                        tunnel: w480 -> [w486 _]
                        tunnel: w477 -> [_ w494]
                        tunnel: w462 -> [_ w491]
                        frame False {
                          # "No new file - use old file name"
                        }
                        frame True {
                          # "new multi file name required"
                          n110 = Unbundle By Name(w491) -> ("serno_digits"=w490:i32, "fixed_width"=w489:bool, "new_file_mode"=w488:u16, "time_format_string"=w487:string)
                          n111 = Select(t=w490, s=w489, f=0) -> (s? t:f=w492:i32)
                          n112 = call "ex_BuildFilepath.vi"("serial digits"=w492, "serial num"=w496, "time format string"=w487, "naming mode"=w488, "name base"=w494) -> ("built name"=w495:path)  [unwired: 1 in, 5 out]
                        }
                      }
                      n113 = Unbundle By Name(w470) -> ("Flags"=w475:T4)
                      n114 = Bundle By Name(cluster=w475, "col headings always?"=w473) -> (w476:T4)
                      n115 = Unbundle By Name(w462) -> ("File refnum"=w466:refnum<file>, "overwrite_mode_multi"=w459:T6, "overwrite_mode"=w458:T1, "File Dialog"=w468:bool, "Description Out"=w444:string, "Comment Out"=w443:string, "Simulate Non-First Call"=w445:bool)
                      n116 = Bundle By Name(cluster=w470, "origin time"=w463, "Flags"=w476, "Flags.x_columns"=w461) -> (w460:T3)
                      n117 = Or(x=w453, y=w471) -> (x .or. y?=w472:bool)
                      n118 = And(x=w468, y=w472) -> (x .and. y?=w457:bool)
                      n119 = call "ex_WriteDataTDMS.vi"("file path"=w456, "first call"=w453, "Lock file"=w442, "Signals"=w465, "overwrite_mode_multi"=w459, "overwrite_mode"=w458, "error in (no error)"=w464, "file dialog?"=w457, "Description"=w444, "multi_file"=w454, "Comment"=w443, "new file?"=w455, "Simulate Non-First Call"=w445, "file params"=w460, "append info in"=w447, "DAQmx Task"=w446) -> ("operator cancelled?"=w450:bool, "file path out"=w452:path, "bytes written"=w449:i32, "append info out"=w448:T13, "error out"=w451:errorcluster)  [unwired: 7 in]
                    }
                    frame True {
                      w511 = FALSE  # operator cancelled?
                      w515 = 0  # mark after write (bytes)
                      w513 = 0  # 1st Serial #
                      # "True: First enabled call"
                      n120 = for {
                        tunnel: w508 -> [w517] mode=indexing
                        tunnel: [w516] -> w507 mode=indexing
                        n121 = Unbundle By Name(w517) -> ("Start Timestamp"=w516:timestamp)
                      }
                      n122 = Array Max & Min(array=w507) -> (min value=w505:timestamp)  [unwired: 3 out]
                      n123 = Bundle By Name(cluster=w506, "origin time"=w505) -> (w504:T11)
                    }
                  }
                }
                frame condition #1 {
                  n124 = Unbundle By Name(w525) -> ("File refnum"=w524:refnum<file>)
                }
              }
            }
          }
          n125 = case shown="True" w99 {
            tunnel: [FALSE ("Ask each iteration") "Ask each iteration"] -> w98
            frame False {
              # "Otherwise, after ex_subFileWriter.vi is invoked for the first time, set \"1st\" to false."
            }
            frame True {
              # "If \"Ask user to choose file\" is checked and \"Ask each iteration\" is selected by user, then each invocation of ex_subFileWrite.vi is treated as the first time's invocation."
            }
          }
          n126 = case shown="True" w98 {
            tunnel: w97 -> [w137 _]
            tunnel: [w137 FALSE ("operator cancelled?")] -> w96
            frame False {
            }
            frame True {
            }
          }
        }
        n127 = local write "File refnum"(w88) -> ()
        n128 = local write "1st"(w80) -> ()
        "previous path" <- w82
      }
    }
  }
  "error out" <- w31
  "File Path out" <- w30
  n129 = Not A Number/Path/Refnum?(number/path/refnum=w30) -> (NaN/Path/Refnum?=w42:bool)
  n130 = Not(x=w42) -> (.not. x?=w41:bool)
  n131 = And(x=w41, y="Enable") -> (x .and. y?=→"Saving Data":bool)
